vi "HTTPMethod_PostData.vi"(7 "LabVIEW Web Service Request":refnum<class "Web Request.lvclass">) -> (3 "ID":cluster{"Nom":string, "Age":u8})   [LabVIEW 2020]
uses:
  <vilib>/wsapi/Web Request.lvclass
panel:
  out "Value":string[](array[string])
  out "Key":string[](array[string])
  out "postdata":string
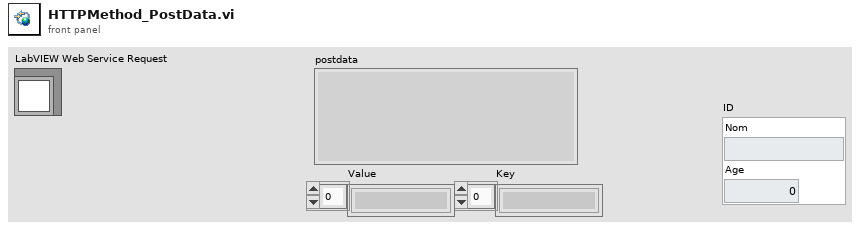
[diagram p1: front panel]
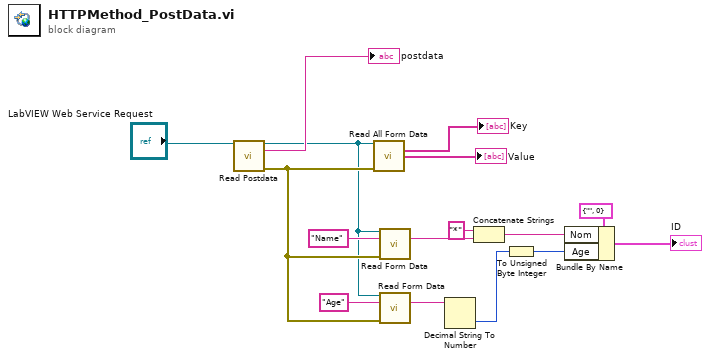
[diagram p0: block diagram]
diagram:
  n1 = call <vilib>:"Read Postdata.vi"("LabVIEW Web Service Request"="LabVIEW Web Service Request") -> ("LabVIEW Web Service Request out"=w1:refnum<class "Web Request.lvclass">, "postdata"=→"postdata":string, "error out"=w5:errorcluster)  [unwired: 12 in]
  n2 = call <vilib>:"Read All Form Data.vi"("LabVIEW Web Service Request"=w1, "error in (no error)"=w5) -> ("Key"=→"Key":string[], "Value"=→"Value":string[])  [unwired: 9 in, 3 out]
  n3 = call <vilib>:"Read Form Data.vi"("LabVIEW Web Service Request"=w1, "key"="Name", "error in (no error)"=w5) -> ("value"=w9:string)  [unwired: 9 in, 3 out]
  n4 = call <vilib>:"Read Form Data.vi"("LabVIEW Web Service Request"=w1, "key"="Age", "error in (no error)"=w5) -> ("value"=w4:string)  [unwired: 9 in, 3 out]
  n5 = Decimal String To Number(string=w4) -> (number=w3:i32)  [unwired: 2 in, 1 out]
  n6 = Concatenate Strings("*" ("string"), w9) -> (w8:string)
  n7 = To Unsigned Byte Integer(number=w3) -> (unsigned 8bit integer=w2:u8)
  n8 = Bundle By Name(cluster=cluster{"Nom":string, "Age":u8} {"Nom"="", "Age"=0} ("ID"), "Nom"=w8, "Age"=w2) -> (→"ID":cluster{"Nom":string, "Age":u8})
